vi "BW-convert.vi"(11 "Input pixel":u32) -> (3 "Output pixel":dbl)   [LabVIEW 2021]
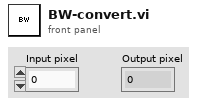
[diagram p1: front panel]
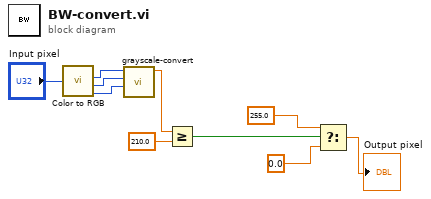
[diagram p0: block diagram]
diagram:
  n1 = call <vilib>:"Color to RGB.vi"("Color"="Input pixel") -> ("R"=w6:u8, "G"=w7:u8, "B"=w8:u8)  [unwired: 1 out]
  n2 = call "grayscale-convert.vi"("B"=w8, "G"=w7, "R"=w6) -> ("Output pixel"=w10:dbl)  [unwired: 8 in]
  n3 = Greater Or Equal?(x=w10, y=210.0) -> (x >= y?=w1:bool)
  n4 = Select(t=255.0, s=w1, f=0.0) -> (s? t:f=→"Output pixel":dbl)
